vi "Bind To Name - Class - Type Name Is Fully Qualified Class Name.vi"() -> ()   [LabVIEW 2017, in "Default Serialization Binder Tests.lvlib"]
uses:
  Default Serialization Binder Tests.lvlib
  Default Serialization Binder/Default Serialization Binder.lvclass
  Class/Class.lvclass
  <vilib>/addons/_JKI Toolkits/Caraya/classes/Assert/Assert Equal Value_Variant.vi
  <vilib>/addons/_JKI Toolkits/Caraya/classes/Test/Test.lvclass
  <vilib>/addons/_JKI Toolkits/Caraya/classes/Assert/Assert.lvclass
panel:
  out "error out":errorcluster
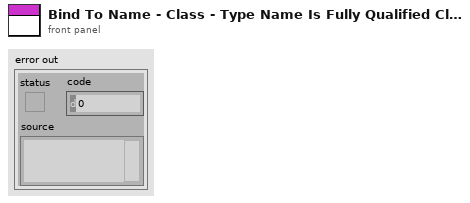
[diagram p1: front panel]
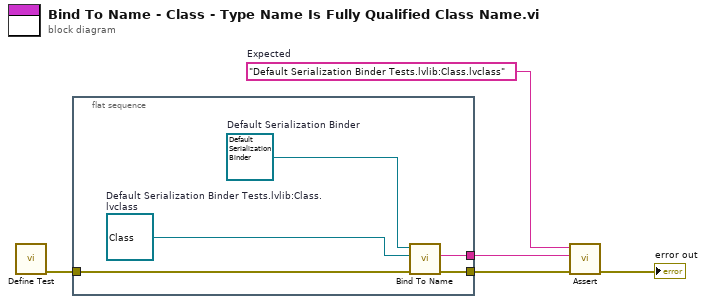
[diagram p0: block diagram]
diagram:
  w1 = "Default Serialization Binder Tests.lvlib:Class.lvclass"  # Expected
  n1 = call <vilib>:"Define Test.vi"() -> ("error out"=w4:errorcluster)  [unwired: 11 in]
  n2 = flat-sequence {
    tunnel: w4 -> [w8]
    tunnel: [w7] -> w3
    tunnel: [w6] -> w2
    frame #0 {
      w9 = refnum<class "Class.lvclass"> refnum  # Default Serialization Binder Tests.lvlib:Class.lvclass
      w10 = refnum<class "Default Serialization Binder.lvclass"> refnum  # Default Serialization Binder
      n3 = call-dynamic "Bind To Name.vi"("error in (no error)"=w8, "Type"=w9, "Default Serialization Binder in"=w10) -> ("error out"=w7:errorcluster, "Type Name"=w6:string)  [unwired: 6 in, 1 out]
    }
  }
  n4 = call-poly <vilib>:"Assert.vi"("error in (no error)"=w3, "Y"=w2, "X"=w1) -> ("error out"=→"error out":errorcluster)  [unwired: 8 in]
